vi "Parse FPGA Bitfile.vi"(8 "error in (no error)":errorcluster, 10 "fgpa cd ref":T1=18446744073709551615 format="%.0x", 11 "Path":path) -> (0 "error out":errorcluster, 2 "fpga resources":T2[](array[typedef]) {"fgpa cd ref" format="%.0x"; "reserver ref" format="%.0x"})   [LabVIEW 2016, in "FPGA Addon System Explorer.lvlib"]
uses:
  FPGA Addon System Explorer.lvlib
  fpga resource.ctl
  Channel Type.ctl
  <vilib>/NI Veristand/Custom Device API/Custom Device Item Ref.ctl
  <vilib>/rvi/ClientSDK/Host Interface/DMA/public/niFpgaDmaChannelVisibilityFilter.ctl
  <vilib>/rvi/ClientSDK/Core/ModuleGeneration/CommunicationInterfaceUtility/niFpgaDmaChannelImplementation.ctl
  <vilib>/NI VeriStand/Custom Device API/Custom Device API.lvlib
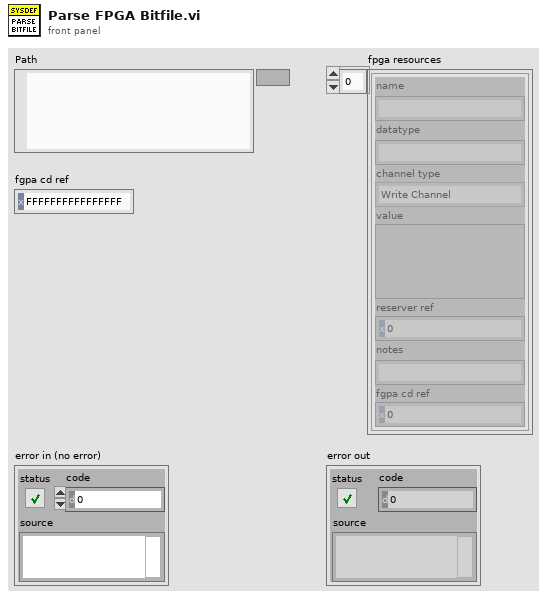
[diagram p1: front panel]
types:
  T1 = typedef "Custom Device API.lvlib/Custom Device Item Ref.ctl" = u64
  T2 = typedef "FPGA Addon System Explorer.lvlib/fpga resource.ctl" = cluster{"name":string, "datatype":string, "channel type":T3, "value":variant, "reserver ref":T1, "notes":string, "fgpa cd ref":T1}
  T3 = typedef "FPGA Addon System Explorer.lvlib/Channel Type.ctl" = enum16{"Write Channel", "Read Channel", "Write Waveform", "Read Waveform"}
  T4 = typedef "niFpgaDmaChannelVisibilityFilter.ctl" = enum16{"All", "UserVisible"}
  T5 = typedef "niFpgaDmaChannelImplementation.ctl" = enum16{"niFpgaTargetToHost", "niFpgaHostToTarget", "niFpgaPeerToPeerWriter", "niFpgaPeerToPeerReader", "niCoreTargetToHost", "niCoreHostToTarget"}
  T6 = typedef "Fifo_DMA_Config.ctl" = cluster{"Name":string, "Depth":u32, "Write? (Deprecated:Use Implementation)":bool, "Physical Channel":u32, "Base Address":u32, "Data Width":u32, "Data Type":T7, "FXP Properties":variant, "Write Window Address":u32, "Implementation":T5, "Control Set":u32}
  T7 = typedef "niFpgaDataTypeControl.ctl" = enum32{"Boolean", "I8", "I16", "I32", "I64", "U8", "U16", "U32", "U64", "FXP", "CustomControl", "SGL"}
  T8 = typedef "niFpgaBitfileStructure_VI.ctl" = cluster{"Name":string, "RegisterMap":T9[], "Icon":T14}
  T9 = typedef "nirviControlStructure.ctl" = cluster{"Name":string, "Hidden":bool, "Indicator":bool, "Flattened Type":string, "Grouping":cluster{"Grouped":bool, "Member Names":string[], "Member IDs":u32[]}, "Address":u32, "Size":u32, "Class":u32, "Internal":bool, "Typedef":T10, "ID":u32, "Bidirectional":bool, "Synchronous":bool, "Mechanical Action":T11, "Sub Controls":T12[], "Access May Timeout":bool, "Register Node":bool}
  T10 = typedef "nirviTypdefDescription.ctl" = cluster{"Typedef":bool, "Path":path}
  T11 = typedef "nirviMechanicalAction.ctl" = enum8{"Switch When Pressed", "Switch When Released", "Switch Until Released", "Latch When Pressed", "Latch When Released", "Latch Until Released"}
  T12 = typedef "nirviSubControlStructure.ctl" = cluster{"Name":string, "flattened Type":string, "Cluster Information":T13, "Typedef":T10}
  T13 = typedef "nirviClusterElementControl.ctl" = cluster{"Name Hierarchy":string[], "Item Order":u32[]}
  T14 = typedef "imagedata.ctl" = cluster{"image type":i32, "image depth":i32, "image":u8[], "mask":u8[], "colors":u32[], "Rectangle":cluster{"left":i16, "top":i16, "right":i16, "bottom":i16}}
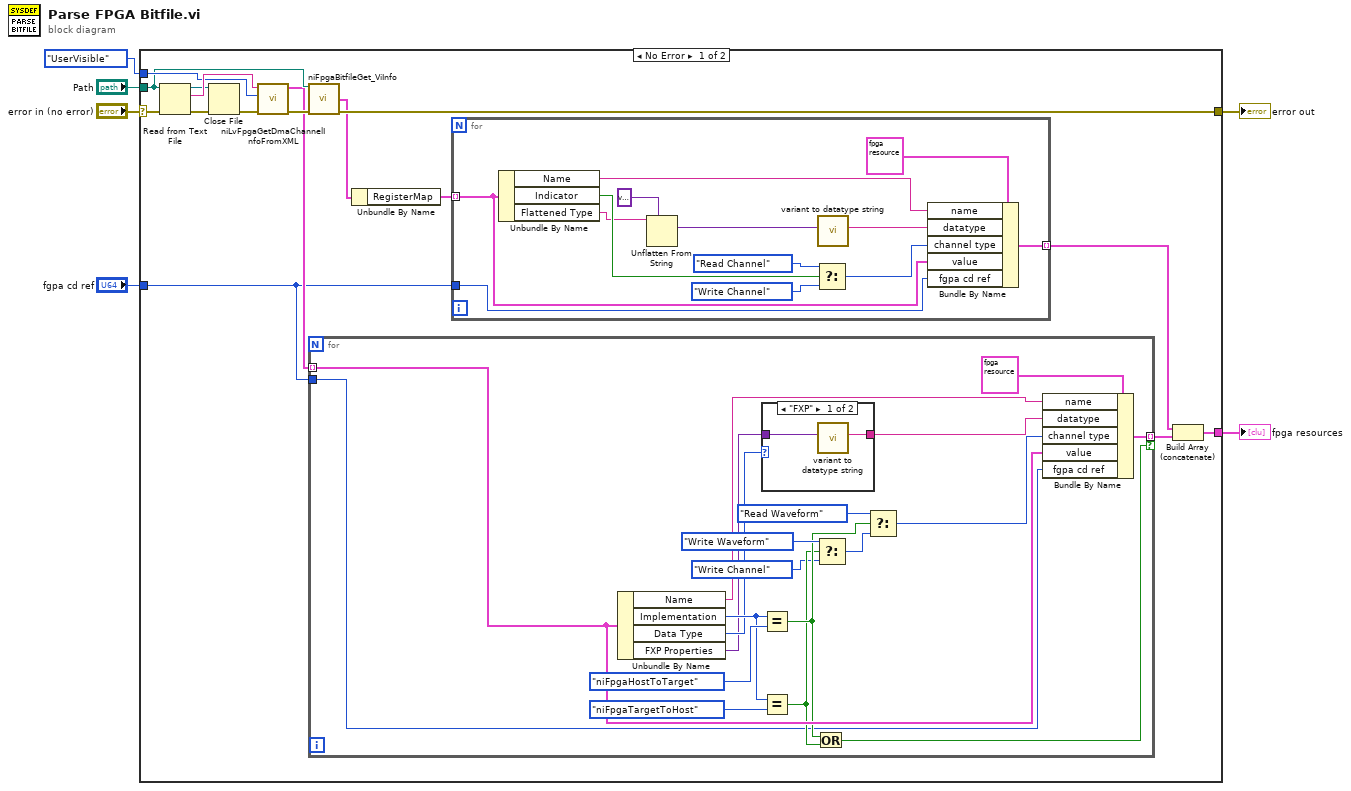
[diagram p0: block diagram]
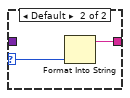
[diagram p2: hidden frame]
diagram:
  n1 = case shown="No Error" "error in (no error)" {
    selector: "error in (no error)" -> [w18 w59]
    tunnel: [w14 w59] -> w5
    tunnel: "Path" -> [w16 _]
    tunnel: niFpgaDmaChannelVisibilityFilter."UserVisible" ("DMA Channel Filter") -> [w17 _]
    tunnel: [w8 _] -> w2
    tunnel: "fgpa cd ref" -> [w7 _]
    frame No Error {
      n2 = Read from Text File(file (use dialog)=w16, error in=w18) -> (refnum out=w21:refnum<file>, text=w22:string, error out=w20:errorcluster)  [unwired: 3 out]
      n3 = Close File(refnum=w21, error in=w20) -> (error out=w19:errorcluster)  [unwired: 1 out]
      n4 = call <resource>:"niLvFpgaGetDmaChannelInfoFromXML.vi"("error in (no error)"=w19, "DMA Channel Filter"=w17, "XML String in"=w22) -> ("error out"=w15:errorcluster, "DMA configuration array"=w13:T6[])  [unwired: 7 out]
      n5 = call <vilib>:"niFpgaBitfileGet_ViInfo.vi"("bitfile path"=w16, "error in (no error)"=w15) -> ("vi info"=w12:T8, "error out"=w14:errorcluster)  [unwired: 1 in, 11 out]
      n6 = for {
        tunnel: w13 -> [w52] mode=indexing
        tunnel: [w45] -> w9 mode=indexing if=w42
        tunnel: w7 -> [w36]
        n7 = Unbundle By Name(w52) -> ("Name"=w53:string, "Implementation"=w49:T5, "Data Type"=w40:T7, "FXP Properties"=w37:variant)
        n8 = case shown="\"FXP\"" w40 {
          selector: w40 -> [_ w58]
          tunnel: [w55 w57] -> w39
          tunnel: w37 -> [w56 _]
          frame "FXP" {
            n9 = call "variant to datatype string.vi"("Variant"=w56) -> ("datatype string"=w55:string)  [unwired: 9 in, 1 out]
          }
          frame Default {
            n10 = Format Into String(w58) -> (resulting string=w57:string)  [unwired: 3 in, 1 out]
          }
        }
        n11 = Equal?(x=w49, y=niFpgaDmaChannelImplementation."niFpgaHostToTarget") -> (x = y?=w44:bool)
        n12 = Equal?(x=w49, y=niFpgaDmaChannelImplementation."niFpgaTargetToHost") -> (x = y?=w43:bool)
        n13 = Or(x=w44, y=w43) -> (x .or. y?=w42:bool)
        n14 = Select(t=Channel_Type."Write Waveform" ("type"), s=w43, f=Channel_Type."Write Channel") -> (s? t:f=w47:T3)
        n15 = Select(t=Channel_Type."Read Waveform", s=w44, f=w47) -> (s? t:f=w41:T3)
        n16 = Bundle By Name(cluster=T2 {"name"="", "datatype"="", "channel type"=enum."Write Channel", "value"=variant, "reserver ref"=0, "notes"="", "fgpa cd ref"=0} ("FPGA Resource"), "name"=w53, "datatype"=w39, "channel type"=w41, "value"=w52, "fgpa cd ref"=w36) -> (w45:T2)
      }
      n17 = Unbundle By Name(w12) -> ("RegisterMap"=w11:T9[])
      n18 = for {
        tunnel: w11 -> [w24] mode=indexing
        tunnel: [w25] -> w10 mode=indexing
        tunnel: w7 -> [w23]
        n19 = Unbundle By Name(w24) -> ("Name"=w34:string, "Indicator"=w33:bool, "Flattened Type"=w29:string)
        n20 = Unflatten From String(type=variant, binary string=w29) -> (value=w27:variant)  [unwired: 3 in, 2 out]
        n21 = Select(t=Channel_Type."Read Channel" ("type"), s=w33, f=Channel_Type."Write Channel") -> (s? t:f=w30:T3)
        n22 = call "variant to datatype string.vi"("Variant"=w27) -> ("datatype string"=w26:string)  [unwired: 9 in, 1 out]
        n23 = Bundle By Name(cluster=T2 {"name"="", "datatype"="", "channel type"=enum."Write Channel", "value"=variant, "reserver ref"=0, "notes"="", "fgpa cd ref"=0} ("FPGA Resource"), "name"=w34, "datatype"=w26, "channel type"=w30, "value"=w24, "fgpa cd ref"=w23) -> (w25:T2)
      }
      n24 = Build Array (concatenate)(w10, w9) -> (w8:T2[])
    }
    frame Error {
    }
  }
  "error out" <- w5
  "fpga resources" <- w2
